vi "Fit Image to Ctrl (SubVI).vi"(10 "picture in":picture, 11 "Picture ref in":refnum<vi>) -> ()   [LabVIEW 2014, in "SeqLoop.lvlib" / "Mimico Display.lvlib"]
uses:
  Mimico Display.lvlib
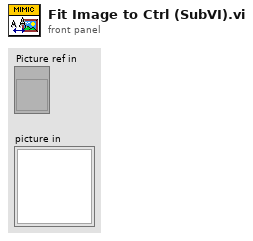
[diagram p1: front panel]
types:
  T1 = typedef "LVBoundsTypeDef.ctl" = cluster{"Width":u32, "Height":u32}
  T2 = typedef "imagedata.ctl" = cluster{"image type":i32, "image depth":i32, "image":u8[], "mask":u8[], "colors":u32[], "Rectangle":cluster{"left":i16, "top":i16, "right":i16, "bottom":i16}}
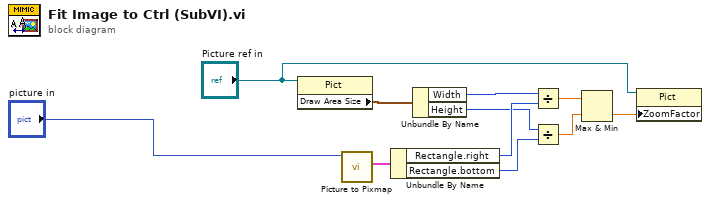
[diagram p0: block diagram]
diagram:
  n1 = property class="Pict"(reference="Picture ref in") -> ("Draw Area Size"=w4:T1)  [unwired: 1 in, 2 out]
  n2 = call <vilib>:"Picture to Pixmap.vi"("picture"="picture in") -> ("image data"=w10:T2)  [unwired: 9 in, 1 out]
  n3 = Unbundle By Name(w10) -> ("Rectangle.right"=w7:i16, "Rectangle.bottom"=w8:i16)
  n4 = Unbundle By Name(w4) -> ("Width"=w5:u32, "Height"=w6:u32)
  n5 = Divide(x=w5, y=w7) -> (x/y=w3:dbl)
  n6 = Divide(x=w6, y=w8) -> (x/y=w2:dbl)
  n7 = Max & Min(x=w3, y=w2) -> (min(x,y)=w1:dbl)  [unwired: 1 out]
  n8 = property class="Pict"(reference="Picture ref in", "ZoomFactor"=w1) -> ()  [unwired: 1 in, 2 out]
